vi "Write Run.vi"(10 "Run":refnum<user-event>, 11 "DAQ in":refnum<class "DAQ.lvclass">) -> (3 "DAQ out":refnum<class "DAQ.lvclass">)   [LabVIEW 2011, in "DAQ.lvclass"]
uses:
  DAQ.lvclass
  DAQ.lvclass/DAQ.ctl
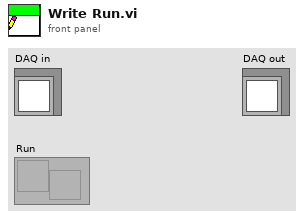
[diagram p1: front panel]
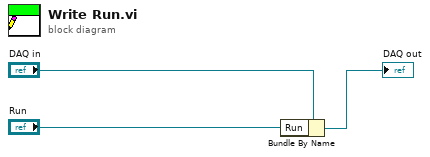
[diagram p0: block diagram]
diagram:
  n1 = Bundle By Name(cluster="DAQ in", "Run"="Run") -> (→"DAQ out":refnum<class "DAQ.lvclass">)
